vi "SD-STR_ASCII-Unicode.vi"(1 "ASCII string":string) -> (0 "unicode string":string)   [LabVIEW 2020]
doc: "This VI converts an ASCII string to a unicode string."
uses:
  kernel32.dll
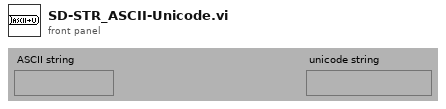
[diagram p1: front panel]
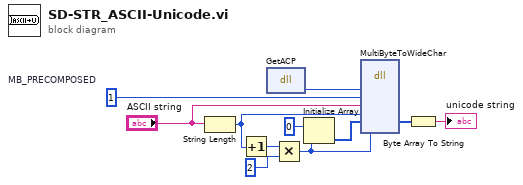
[diagram p0: block diagram]
diagram:
  w10 = u32 1  # MB_PRECOMPOSED
  n1 = String Length(string="ASCII string") -> (length=w3:i32)
  n2 = Increment(x=w3) -> (x+1=w8:i32)
  n3 = dll-call lib="kernel32.dll" fn="GetACP" label="GetACP()"() -> (w1:u32)  [unwired: 3 in, 2 out]
  n4 = Multiply(x=w8, y=2) -> (x*y=w2:i32)
  n5 = Initialize Array(u8 0, w2) -> (w6:u8[])
  n6 = dll-call lib="kernel32.dll" fn="MultiByteToWideChar"("codePage"=w1, "dwFlags"=w10, "lpCStr"="ASCII string", "nChars"=w3, "lpWStr"=w6, "nWStr"=w2) -> ("lpWStr"=w5:u8[])  [unwired: 8 in, 3 out]
  n7 = Byte Array To String(unsigned byte array=w5) -> (string=→"unicode string":string)
